vi "New motor Control integrated remodeled state based.vi"(2 "Error in":errorcluster, 3 "Yaw":dbl, 4 "States":T2) -> (0 "Error out":errorcluster, 1 "Speed and distance cluster":T1)   [LabVIEW 2018]
uses:
  Motor Control/States for motor control.ctl
panel:
  in  "Boolean":bool=TRUE
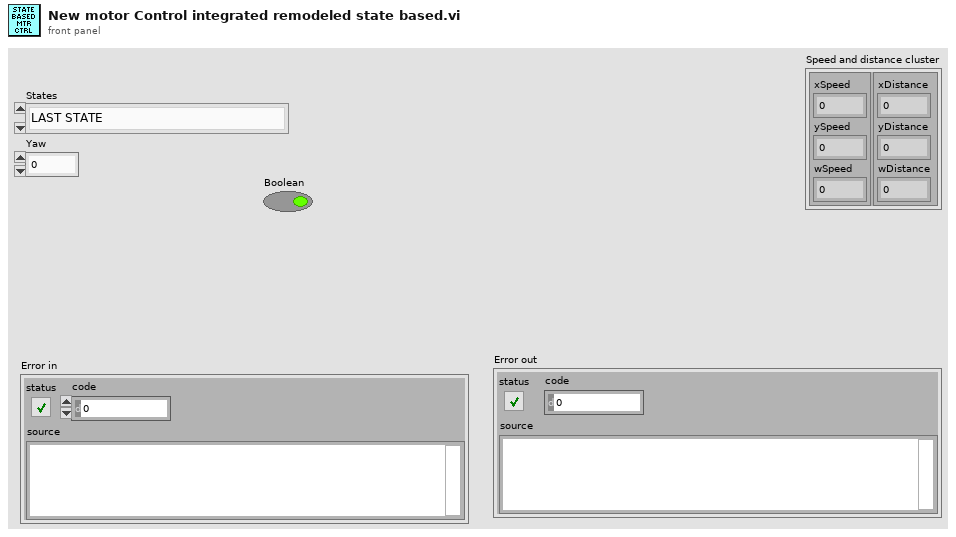
[diagram p1: front panel]
types:
  T1 = cluster{cluster{"xSpeed":dbl, "ySpeed":dbl, "wSpeed":dbl}, cluster{"xDistance":dbl, "yDistance":dbl, "wDistance":dbl}}
  T2 = typedef "States for motor control.ctl" = enum16{"LAST STATE", "STOP", "FORWARD", "BACKWARD", "LEFT", "RIGHT", "RCW", "ACW", "INIT", "RESET ENCODERS"}
  T3 = cluster{"Encoder 0":dbl, "Encoder 1":dbl, "Encoder 2":dbl}
  T4 = cluster{"xTargetSpeed":dbl, "yTargetSpeed":dbl, "wTargetSpeed":dbl}
  T5 = cluster{"Distance M0 ":dbl, "Distance M1 ":dbl, "Distance M2 ":dbl}
  T6 = cluster{"xDistance":dbl, "yDistance":dbl, "wDistance":dbl}
  T7 = cluster{"xSpeed":dbl, "ySpeed":dbl, "wSpeed":dbl}
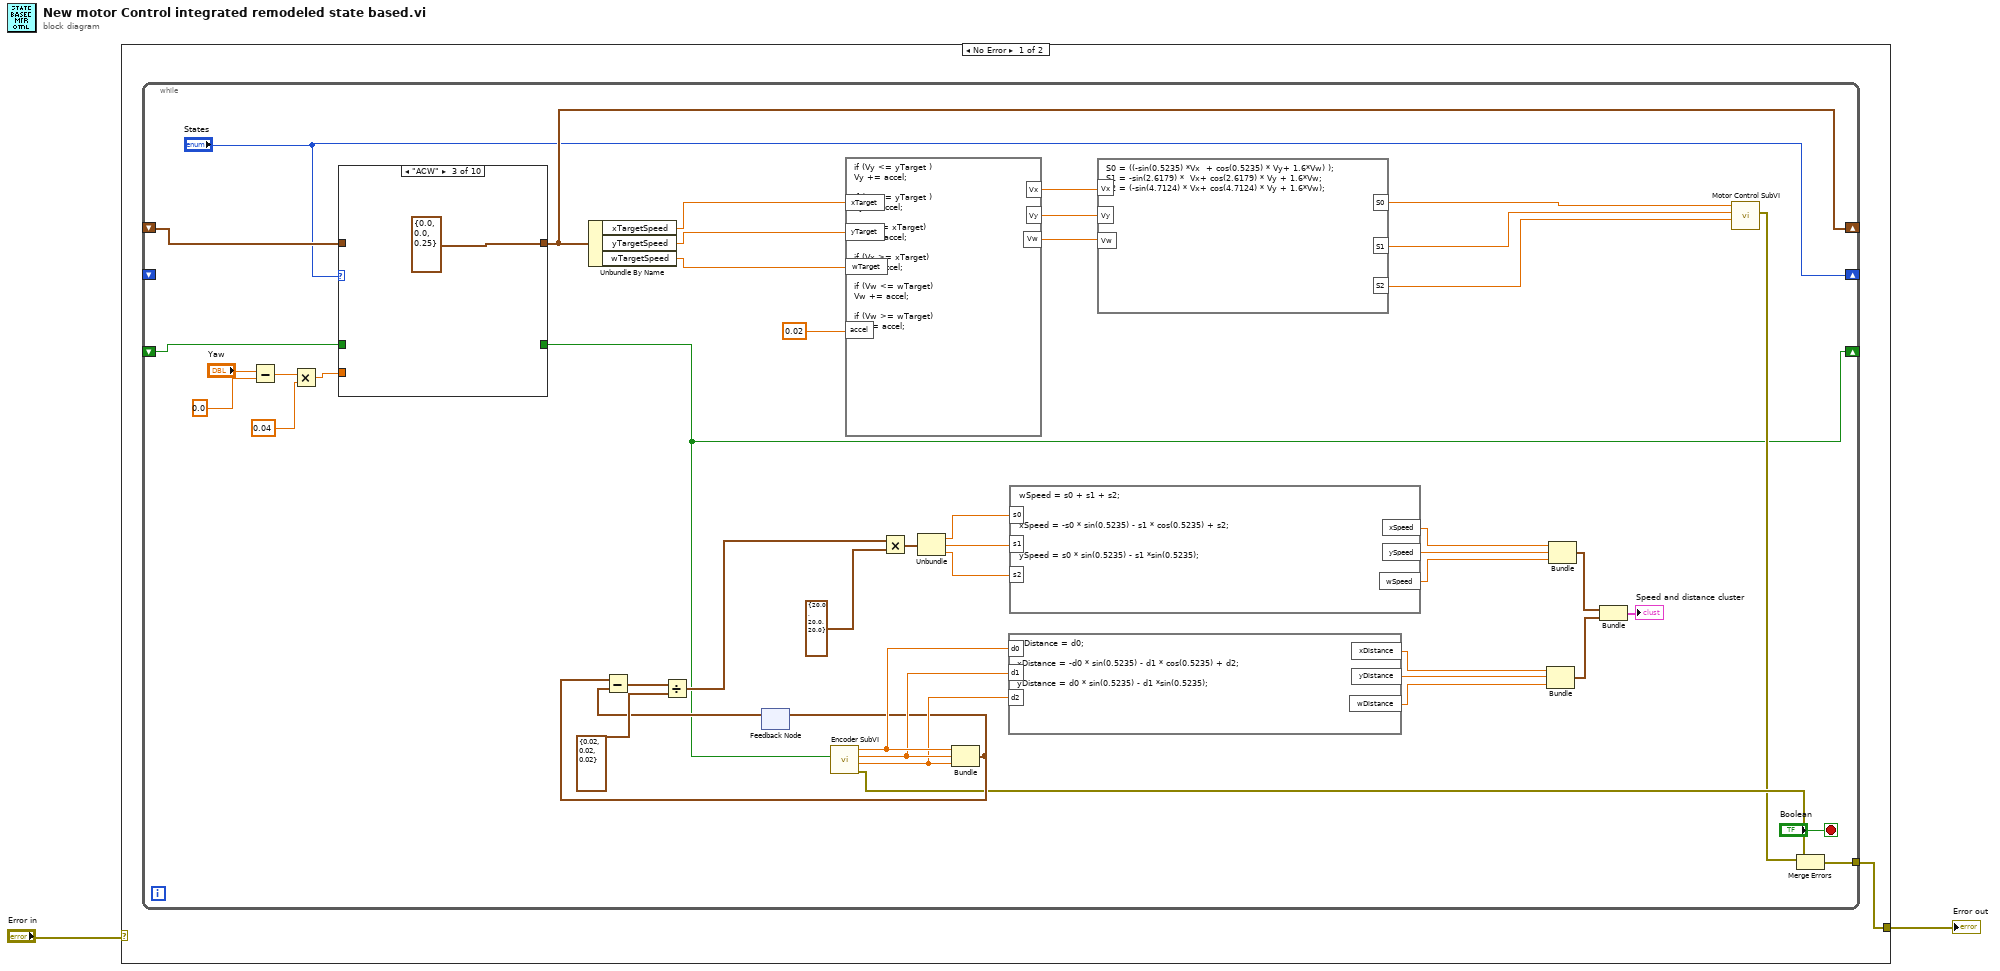
[diagram p0: block diagram]
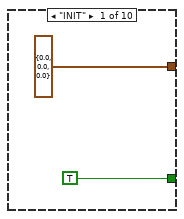
[diagram p2: hidden frame]
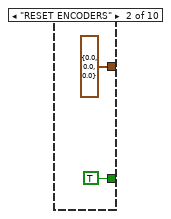
[diagram p3: hidden frame]
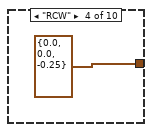
[diagram p4: hidden frame]
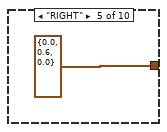
[diagram p5: hidden frame]
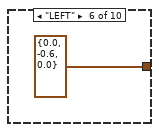
[diagram p6: hidden frame]
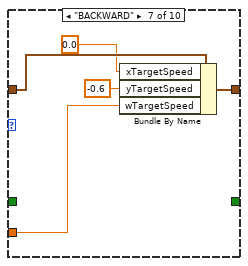
[diagram p7: hidden frame]
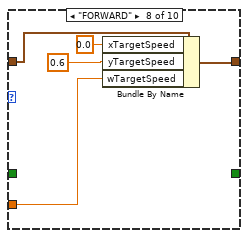
[diagram p8: hidden frame]
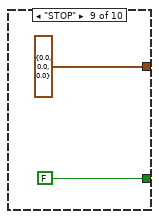
[diagram p9: hidden frame]
diagram:
  n1 = case shown="No Error" "Error in" {
    selector: "Error in" -> [_ w71]
    tunnel: [w3 w71] -> w1
    frame No Error {
      n2 = while {
        shift-right: [w30] -> _
        shift-left: _ -> [w29]
        tunnel: [w24] -> w3
        shift-right: [w23] -> _
        shift-left: _ -> [w22]
        shift-right: ["States"] -> _
        shift-left: _ -> [_]
        stop <- "Boolean" stop-if-true
        n3 = Subtract(x="Yaw", y=0.0) -> (x-y=w7:dbl)
        n4 = Multiply(x=w7, y=0.04) -> (x*y=w5:dbl)
        n5 = case shown="\"ACW\"" "States" {
          tunnel: [T4 {"xTargetSpeed"=0.0, "yTargetSpeed"=0.0, "wTargetSpeed"=0.0} ("Target Speed") T4 {"xTargetSpeed"=0.0, "yTargetSpeed"=0.0, "wTargetSpeed"=0.0} ("Target Speed") T4 {"xTargetSpeed"=0.0, "yTargetSpeed"=0.0, "wTargetSpeed"=0.25} ("Target Speed") T4 {"xTargetSpeed"=0.0, "yTargetSpeed"=0.0, "wTargetSpeed"=-0.25} ("Target Speed") T4 {"xTargetSpeed"=0.0, "yTargetSpeed"=0.6, "wTargetSpeed"=0.0} ("Target Speed") T4 {"xTargetSpeed"=0.0, "yTargetSpeed"=-0.6, "wTargetSpeed"=0.0} ("Target Speed") w62 w65 T4 {"xTargetSpeed"=0.0, "yTargetSpeed"=0.0, "wTargetSpeed"=0.0} ("Target Speed") w70] -> w30
          tunnel: w29 -> [_ _ _ _ _ _ w61 w66 _ w70]
          tunnel: [TRUE ("Reset Encoders") TRUE ("Reset Encoders") _ _ _ _ _ _ FALSE ("Reset Encoders") _] -> w23
          tunnel: w22 -> [_ _ _ _ _ _ _ _ _ _]
          tunnel: w5 -> [_ _ _ _ _ _ w58 w67 _ _]
          frame "INIT" {
          }
          frame "RESET ENCODERS" {
          }
          frame "ACW" {
          }
          frame "RCW" {
          }
          frame "RIGHT" {
          }
          frame "LEFT" {
          }
          frame "BACKWARD" {
            n6 = Bundle By Name(cluster=w61, "xTargetSpeed"=0.0, "yTargetSpeed"=-0.6, "wTargetSpeed"=w58) -> (w62:T4)
          }
          frame "FORWARD" {
            n7 = Bundle By Name(cluster=w66, "xTargetSpeed"=0.0, "yTargetSpeed"=0.6, "wTargetSpeed"=w67) -> (w65:T4)
          }
          frame "STOP" {
          }
          frame "LAST STATE" {
          }
        }
        n8 = Unbundle By Name(w30) -> ("xTargetSpeed"=w12:dbl, "yTargetSpeed"=w11:dbl, "wTargetSpeed"=w10:dbl)
        n9 = feedback #1() -> (w42:T5)  [unwired: 1 in]
        n10 = call "Encoder SubVI.vi"("Reset Encoders"=w23) -> ("error out"=w26:errorcluster, "Distance M2"=w39:dbl, "Distance M1"=w40:dbl, "Distance M0"=w41:dbl)  [unwired: 7 in]
        n11 = formula code="if (Vy <= yTarget )\nVy += accel;\n\nif (Vy >= yTarget )\nVy -= accel;\n\nif(Vx <= xTarget)\nVx += accel;\n\nif (Vx >= xTarget)\nVx -= accel;\n\nif (Vw <= wTarget)\nVw += accel;\n\nif (Vw >= wTarget)\nVw -= accel;"("xTarget"=w12, "yTarget"=w11, "wTarget"=w10, "accel"=0.02 ("input variable")) -> ("Vy"=w15:dbl, "Vx"=w16:dbl, "Vw"=w14:dbl)
        n12 = Bundle("Distance M0"=w41, "Distance M1"=w40, "Distance M2"=w39) -> (w31:T5)  [unwired: 1 in]
        n13 = Subtract(x=w31, y=w42) -> (x-y=w49:T5)
        n14 = Divide(x=w49, y=T3 {"Encoder 0"=0.02, "Encoder 1"=0.02, "Encoder 2"=0.02}) -> (x/y=w35:cluster{dbl, dbl, dbl})
        n15 = feedback-in #1(w31) -> ()
        n16 = Multiply(x=w35, y=cluster{dbl, dbl, dbl} {20.0, 20.0, 20.0}) -> (x*y=w21:cluster{dbl, dbl, dbl})
        n17 = Unbundle(w21) -> (w33:dbl, w44:dbl, w43:dbl)
        n18 = formula code="wDistance = d0;\n\nxDistance = -d0 * sin(0.5235) - d1 * cos(0.5235) + d2;\n\nyDistance = d0 * sin(0.5235) - d1 *sin(0.5235);"("d0"=w41, "d1"=w40, "d2"=w39) -> ("xDistance"=w38:dbl, "wDistance"=w36:dbl, "yDistance"=w37:dbl)
        n19 = formula code="wSpeed = s0 + s1 + s2;\n\n\nxSpeed = -s0 * sin(0.5235) - s1 * cos(0.5235) + s2;\n\n\nySpeed = s0 * sin(0.5235) - s1 *sin(0.5235);"("s0"=w33, "s1"=w44, "s2"=w43) -> ("xSpeed"=w46:dbl, "ySpeed"=w47:dbl, "wSpeed"=w45:dbl)
        n20 = formula code="S0 = ((-sin(0.5235) *Vx  + cos(0.5235) * Vy+ 1.6*Vw) );\nS1 = -sin(2.6179) *  Vx+ cos(2.6179) * Vy + 1.6*Vw;\nS2 = (-sin(4.7124) * Vx+ cos(4.7124) * Vy + 1.6*Vw);"("Vx"=w16, "Vy"=w15, "Vw"=w14) -> ("S0"=w20:dbl, "S1"=w19:dbl, "S2"=w18:dbl)
        n21 = Bundle("xDistance"=w38, "yDistance"=w37, "wDistance"=w36) -> (w28:T6)  [unwired: 1 in]
        n22 = Bundle("xSpeed"=w46, "ySpeed"=w47, "wSpeed"=w45) -> (w17:T7)  [unwired: 1 in]
        n23 = Bundle(w17, w28) -> (→"Speed and distance cluster":T1)  [unwired: 1 in]
        n24 = call "Motor Control SubVI.vi"("Speed M2"=w18, "Speed M1"=w19, "Speed M0"=w20) -> ("Motor Error"=w25:errorcluster)  [unwired: 8 in]
        n25 = Merge Errors(w25, w26) -> (w24:errorcluster)
      }
    }
    frame Error {
    }
  }
  "Error out" <- w1
